vi "DAQList_Set.vi"(8 "error in (no error)":errorcluster, 10 "ColNumbers":i32, 11 "MulticolumnListbox in":refnum<vi>) -> (0 "error out":errorcluster, 3 "MulticolumnListbox out":refnum<vi>)   [LabVIEW 2016]
uses:
  <vilib>/Utility/miscctls.llb/LVRowAndColumnTypeDef.ctl
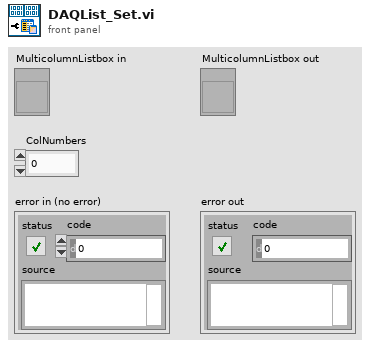
[diagram p1: front panel]
types:
  T1 = cluster{"Font Name":string, "Size":u16, "Bold":bool, "Italic":bool, "Underline":bool, "Strikeout":bool, u32}
  T2 = typedef "LVRowAndColumnTypeDef.ctl" = cluster{"Row":i32, "Column":i32}
  T3 = typedef "LVBoundsTypeDef.ctl" = cluster{"Width":u32, "Height":u32}
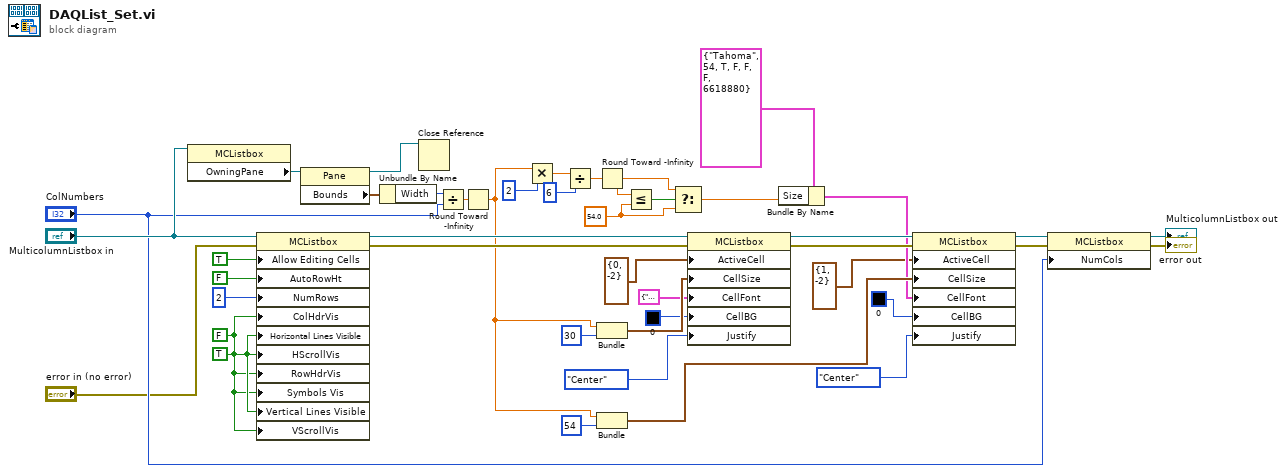
[diagram p0: block diagram]
diagram:
  w22 = 54.0 ("y")
  w5 = TRUE ("Visible Items:Column Headers Visible")
  w4 = FALSE ("Visible Items:Column Headers Visible")
  n1 = property class="MCListbox"(reference="MulticolumnListbox in") -> ("OwningPane"=w15:refnum<vi>)  [unwired: 1 in, 2 out]
  n2 = property class="MCListbox"(reference="MulticolumnListbox in", error in="error in (no error)", "Allow Editing Cells"=TRUE, "AutoRowHt"=FALSE ("Autosizing Row Height"), "NumRows"=u32 2 ("Number of Rows"), "ColHdrVis"=w4, "Horizontal Lines Visible"=w5, "HScrollVis"=w4, "RowHdrVis"=w4, "Symbols Vis"=w4, "Vertical Lines Visible"=w5, "VScrollVis"=w4) -> (reference out=w35:refnum<vi>, error out=w36:errorcluster)
  n3 = property class="Pane"(reference=w15) -> (reference out=w26:refnum<vi>, "Bounds"=w24:T3)  [unwired: 1 in, 1 out]
  n4 = Unbundle By Name(w24) -> ("Width"=w25:u32)
  n5 = Close Reference(reference=w26) -> ()  [unwired: 1 in, 1 out]
  n6 = Divide(x=w25, y="ColNumbers") -> (x/y=w16:dbl)
  n7 = Round Toward -Infinity(1:w16) -> (0:w33:dbl)
  n8 = Multiply(x=w33, y=u32 2) -> (x*y=w18:dbl)
  n9 = Divide(x=w18, y=u32 6) -> (x/y=w21:dbl)
  n10 = Round Toward -Infinity(1:w21) -> (0:w23:dbl)
  n11 = Bundle(w33, "Height"=u32 30) -> (w28:cluster{dbl, "Height":u32})  [unwired: 1 in]
  n12 = Bundle(w33, "Height"=u32 54) -> (w34:cluster{dbl, "Height":u32})  [unwired: 1 in]
  n13 = Less Or Equal?(x=w23, y=w22) -> (x <= y?=w20:bool)
  n14 = Select(t=w23, s=w20, f=w22) -> (s? t:f=w31:dbl)
  n15 = property class="MCListbox"(reference=w35, error in=w36, "ActiveCell"=T2 {"Row"=0, "Column"=-2} ("Active Cell:Active Cell"), "CellSize"=w28, "CellFont"=T1 {"Font Name"="Tahoma", "Size"=14, "Bold"=TRUE, "Italic"=FALSE, "Underline"=FALSE, "Strikeout"=FALSE, 16448250}, "CellBG"=u32 0, "Justify"=enum16{"Left", "Center", "Right"}."Center" ("Active Cell:Cell Justification")) -> (reference out=w37:refnum<vi>, error out=w38:errorcluster)
  n16 = Bundle By Name(cluster=T1 {"Font Name"="Tahoma", "Size"=54, "Bold"=TRUE, "Italic"=FALSE, "Underline"=FALSE, "Strikeout"=FALSE, 6618880}, "Size"=w31) -> (w30:T1)
  n17 = property class="MCListbox"(reference=w37, error in=w38, "ActiveCell"=T2 {"Row"=1, "Column"=-2} ("Active Cell:Active Cell"), "CellSize"=w34, "CellFont"=w30, "CellBG"=u32 0, "Justify"=enum16{"Left", "Center", "Right"}."Center" ("Active Cell:Cell Justification")) -> (reference out=w14:refnum<vi>, error out=w39:errorcluster)
  n18 = property class="MCListbox"(reference=w14, error in=w39, "NumCols"="ColNumbers") -> (reference out=→"MulticolumnListbox out":refnum<vi>, error out=→"error out":errorcluster)
